vi "MaxXY_2018.03.23.vi"(1 "input_xyz_um":T2, 2 "parameters_xy_scan":T1={"image_size_xy_um"=1.0, "frame_size_xy_px"=20, "pixel_dwell_ms"=1.0} {"pixel_dwell_ms" format="%#_13g"; "image_size_xy_um" format="%#_13g"}, 3 "gaussian_fit":bool=TRUE) -> (5 "max_value":dbl, 7 "output_xyz_um":T2, 8 "BestGaussianFit":cluster{dbl[], dbl[]}, 9 "SumXY":cluster{dbl[], dbl[]})   [LabVIEW 2014]
uses:
  <vilib>/Analysis/NI_AALPro.lvlib
  <vilib>/Analysis/NI_AALBase.lvlib
  <vilib>/Analysis/1siggen.llb/Ramp Pattern by Samples.vi
panel:
  out "sum_y":dbl[][](graph)
  out "sum_x":dbl[][](graph)
  out "scan":dbl[][](graph)
  in  "scan_direction":enum32{"0", "1"}(radio) caption="Scan direction:"
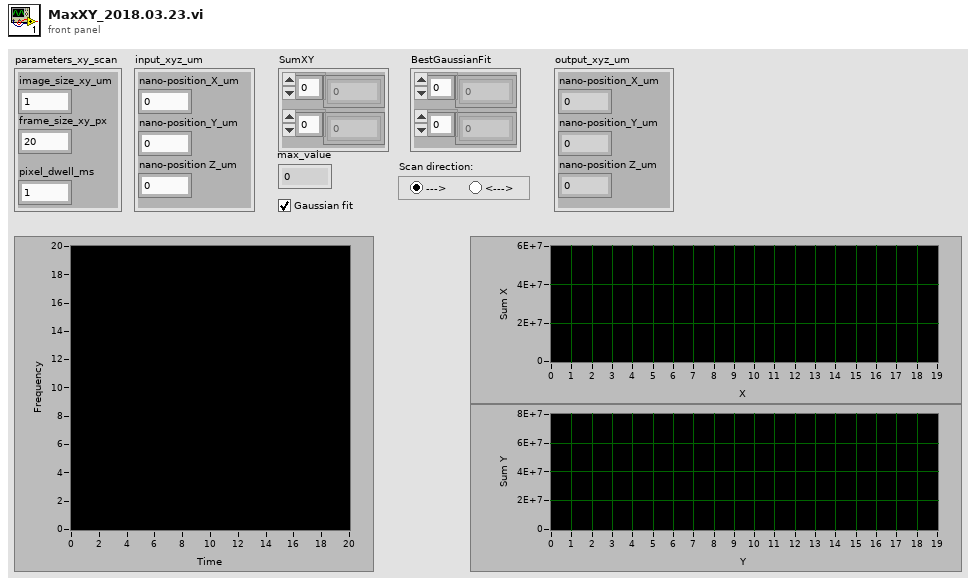
[diagram p1: front panel]
types:
  T1 = cluster{"image_size_xy_um":dbl, "frame_size_xy_px":u32, "pixel_dwell_ms":dbl}
  T2 = cluster{"nano-position_X_um":sgl, "nano-position_Y_um":sgl, "nano-position Z_um":sgl}
  T3 = cluster{"Best Gaussian Fit":dbl[], "Best Gaussian Fit":dbl[]}
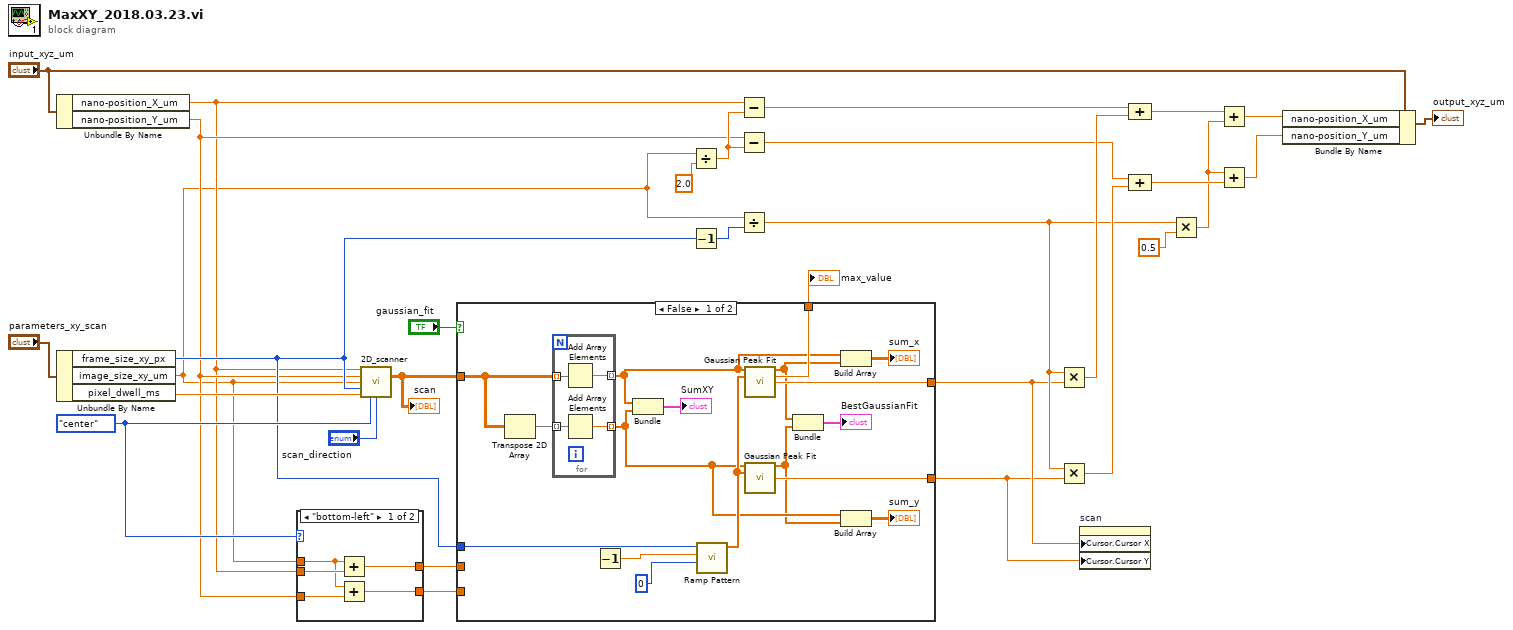
[diagram p0: block diagram]
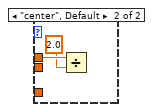
[diagram p2: hidden frame]
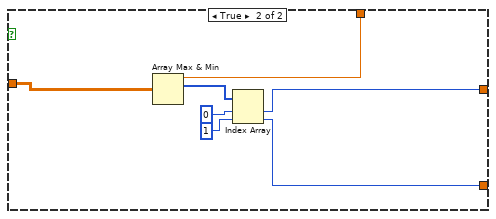
[diagram p3: hidden frame]
diagram:
  w7 = enum32{"bottom-left", "center"}."center" ("pos_start")
  n1 = Unbundle By Name("input_xyz_um") -> ("nano-position_X_um"=w4:sgl, "nano-position_Y_um"=w5:sgl)
  n2 = Unbundle By Name("parameters_xy_scan") -> ("frame_size_xy_px"=w6:u32, "image_size_xy_um"=w3:dbl, "pixel_dwell_ms"=w13:dbl)
  n3 = case shown="\"bottom-left\"" w7 {
    tunnel: w5 -> [w35 _]
    tunnel: w4 -> [w36 _]
    tunnel: w3 -> [w34 w38]
    tunnel: [w33 _] -> w2
    tunnel: [w32 _] -> w1
    frame "bottom-left" {
      n4 = Add(x=w34, y=w36) -> (x+y=w33:dbl)
      n5 = Add(x=w34, y=w35) -> (x+y=w32:dbl)
    }
    frame "center", Default {
      n6 = Divide(x=w38, y=2.0) -> ()  [unwired: 1 out]
    }
  }
  n7 = call "2D_scanner.vi"("pos-start_x"=w4, "pos-start_y"=w5, "image_size_x_um"=w3, "frame_size_x_px"=w6, "pixel_dwell_ms"=w13, "pos_start"=w7, "scan_direction"="scan_direction") -> ("image_out"=w11:dbl[][])  [unwired: 8 in]
  "scan" <- w11
  n8 = case shown="False" "gaussian_fit" {
    tunnel: [w49 w61] -> w9
    tunnel: [w50 w64] -> w10
    tunnel: w11 -> [w54 w63]
    tunnel: [w48 w62] -> w14
    tunnel: w6 -> [w39 _]
    tunnel: w2 -> [_ _]
    tunnel: w1 -> [_ _]
    frame False {
      n9 = Transpose 2D Array(2D array=w54) -> (transposed array=w55:dbl[][])
      n10 = for {
        tunnel: w54 -> [w59] mode=indexing
        tunnel: w55 -> [w58] mode=indexing
        tunnel: [w57] -> w43 mode=indexing
        tunnel: [w56] -> w42 mode=indexing
        n11 = Add Array Elements(numeric array=w59) -> (sum=w57:dbl)
        n12 = Add Array Elements(numeric array=w58) -> (sum=w56:dbl)
      }
      n13 = Decrement() -> (x-1=w53:dbl)  [unwired: 1 in]
      n14 = Bundle(w43, w42) -> (→"SumXY":cluster{dbl[], dbl[]})  [unwired: 1 in]
      n15 = call-poly <vilib>:"Ramp Pattern.vi"("start"=u32 0, "end"=w53, "samples"=w39) -> ("Ramp Pattern"=w51:dbl[])  [unwired: 7 in, 1 out]
      n16 = call <vilib>:"Gaussian Peak Fit.vi"("Y"=w43, "X"=w51) -> ("Best Gaussian Fit"=w41:dbl[], "amplitude"=w48:dbl, "center"=w50:dbl)  [unwired: 7 in, 4 out]
      n17 = call <vilib>:"Gaussian Peak Fit.vi"("Y"=w42, "X"=w51) -> ("Best Gaussian Fit"=w40:dbl[], "center"=w49:dbl)  [unwired: 7 in, 5 out]
      n18 = Bundle("Best Gaussian Fit"=w41, "Best Gaussian Fit"=w40) -> (→"BestGaussianFit":T3)  [unwired: 1 in]
      n19 = Build Array(w43, w41) -> (→"sum_x":dbl[][])
      n20 = Build Array(w42, w40) -> (→"sum_y":dbl[][])
    }
    frame True {
      n21 = Array Max & Min(array=w63) -> (max value=w62:dbl, max index (indices)=w65:i32[])  [unwired: 2 out]
      n22 = Index Array(array=w65, index #1=0 ("index"), index #2=1 ("index")) -> (element #1=w64:i32, element #2=w61:i32)
    }
  }
  "max_value" <- w14
  n23 = Divide(x=w3, y=2.0) -> (x/y=w27:dbl)
  n24 = Decrement(x=w6) -> (x-1=w25:u32)
  n25 = Subtract(x=w4, y=w27) -> (x-y=w26:dbl)
  n26 = Subtract(x=w5, y=w27) -> (x-y=w18:dbl)
  n27 = Divide(x=w3, y=w25) -> (x/y=w24:dbl)
  n28 = Multiply(x=w24, y=w10) -> (x*y=w29:dbl)
  n29 = Multiply(x=w24, y=w9) -> (x*y=w31:dbl)
  n30 = property on="scan" class="IntGraph (strict)"("Cursor.Cursor X"=w10, "Cursor.Cursor Y"=w9) -> ()  [unwired: 2 in, 2 out]
  n31 = Compound Arithmetic op=ADD(w26, w29) -> (w21:dbl)
  n32 = Compound Arithmetic op=ADD(w18, w31) -> (w30:dbl)
  n33 = Multiply(x=w24, y=0.5) -> (x*y=w22:dbl)
  n34 = Add(x=w21, y=w22) -> (x+y=w17:dbl)
  n35 = Add(x=w22, y=w30) -> (x+y=w16:dbl)
  n36 = Bundle By Name(cluster="input_xyz_um", "nano-position_X_um"=w17, "nano-position_Y_um"=w16) -> (→"output_xyz_um":T2)
